vi "Main.vi"() -> ()   [LabVIEW 2018, in "Launcher Main Module.lvlib"]
doc: "This template is based off of the Queued Message Handler design pattern and the Queued Message Handler project template that ships with LabVIEW.\n\nThe main difference is that the queue is private to this module and communication between modules is performed via Broadcast and Request events.\n\nRequest events are wrapped in public API methods and are handled in the Event Handling Loop (EHL) of this VI. Any module can register for Broadcast events sent by this module. The EHL generates messages based on user interface actions.\n\nThe Message Handling Loop (MHL) processes messages generated by the EHL, or by other messages. The messages are string values, so new messages can be added easily to the Message Cases case structure in the MHL. Each message cluster can also provide an optional value for Message Data, which is a variant that can be converted to whatever message-specific data is required.\n_____\nBased on Delacor QMH Project Template 4.2.1.64."
uses:
  Launcher Main Module.lvlib
  <vilib>/Delacor/Delacor QMH/Libraries/Module Admin_class/Delacor_lib_QMH_Module Admin.lvclass
  Module_Controls/Test_Command.ctl
  Module Data--cluster.ctl
  Stop Argument--cluster.ctl
  <vilib>/Delacor/Delacor QMH/Libraries/Message Queue_class/Delacor_lib_QMH_Message Queue.lvclass/Delacor_lib_QMH_Message Queue.ctl
  <vilib>/Delacor/Delacor QMH/Libraries/Module Admin_class/Delacor_lib_QMH_Module Admin.lvclass/Delacor_lib_QMH_Module Admin.ctl
  Module_Controls/Test_Response.ctl
  <vilib>/Utility/miscctls.llb/LVPointTypeDef.ctl
  <vilib>/Delacor/Delacor QMH/Libraries/Message Queue_class/Delacor_lib_QMH_Enqueue Message (Single).vi
  <vilib>/Delacor/Delacor QMH/Libraries/Module Admin_class/Delacor_lib_QMH_Get External Launch.vi
  <vilib>/Utility/error.llb/Error Cluster From Error Code.vi
  <vilib>/ErrorRing/Error Ring.xnode
  <vilib>/Delacor/Delacor QMH/Libraries/Message Queue_class/Delacor_lib_QMH_Message Queue.lvclass
  TCP_Read/TCP_Read.lvlib
  TCP_Write/TCP_Write.lvlib
  TestStand_Control/TestStand_Control.lvlib
panel:
  out "TS_Status":string
  out "command":T1
  out "User_Commands":string
  out "error out":errorcluster
  in  "Module Admin":refnum<class "Delacor_lib_QMH_Module Admin.lvclass">
  out "Status":string
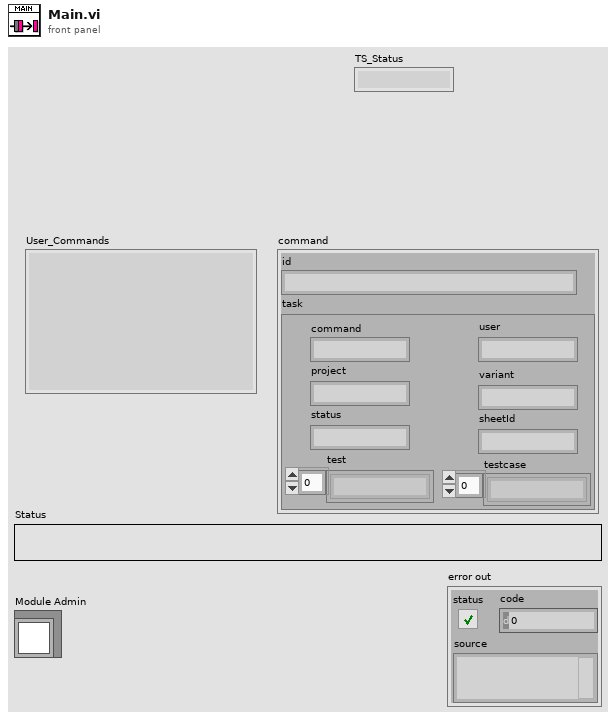
[diagram p1: front panel]
types:
  T1 = typedef "Launcher Main Module.lvlib/Test_Command.ctl" = cluster{"id":string, "task":cluster{"command":string, "project":string, "status":string, "sheetId":string, "test":string[], "user":string, "variant":string, "testcase":string[]}}
  T2 = typedef "Launcher Main Module.lvlib/Request Events--cluster.ctl" = cluster{"Stop Module":refnum<user-event>, "Show Panel":refnum<user-event>, "Hide Panel":refnum<user-event>, "Get Module Execution Status":refnum<user-event>, "Show Diagram":refnum<user-event>}
  T3 = typedef "TestStand_Control.lvlib/Broadcast Events--cluster.ctl" = cluster{"Module Did Init":refnum<user-event>, "Status Updated":refnum<user-event>, "Error Reported":refnum<user-event>, "Module Did Stop":refnum<user-event>, "Update Module Execution Status":refnum<user-event>, "Status":refnum<user-event>}
  T4 = typedef "TCP_Write.lvlib/Broadcast Events--cluster.ctl" = cluster{"Module Did Init":refnum<user-event>, "Status Updated":refnum<user-event>, "Error Reported":refnum<user-event>, "Module Did Stop":refnum<user-event>, "Update Module Execution Status":refnum<user-event>}
  T5 = typedef "TCP_Read.lvlib/Broadcast Events--cluster.ctl" = cluster{"Module Did Init":refnum<user-event>, "Status Updated":refnum<user-event>, "Error Reported":refnum<user-event>, "Module Did Stop":refnum<user-event>, "Update Module Execution Status":refnum<user-event>, "User_Commands":refnum<user-event>}
  T6 = typedef "Launcher Main Module.lvlib/Module Data--cluster.ctl" = cluster{"Status":string}
  T7 = enum32{"invalid lock state", "Not Locked", "Locked (No Password)", "Password-protected"}
  T8 = typedef "Launcher Main Module.lvlib/Stop Argument--cluster.ctl" = cluster{"Origin":string, "Exit via Stop Module Req?":bool, "Wait for Module to stop?":bool}
  T9 = typedef "Launcher Main Module.lvlib/Test_Response.ctl" = cluster{"id":string, "updates":cluster{"status":string}, "command":string, "project":string, "variant":string, "user":string}
  T10 = typedef "LVPointTypeDef.ctl" = cluster{"Horizontal":i16, "Vertical":i16}
  T11 = enum32{"Invalid", "Standard", "Closed", "Hidden", "Minimized", "Maximized"}
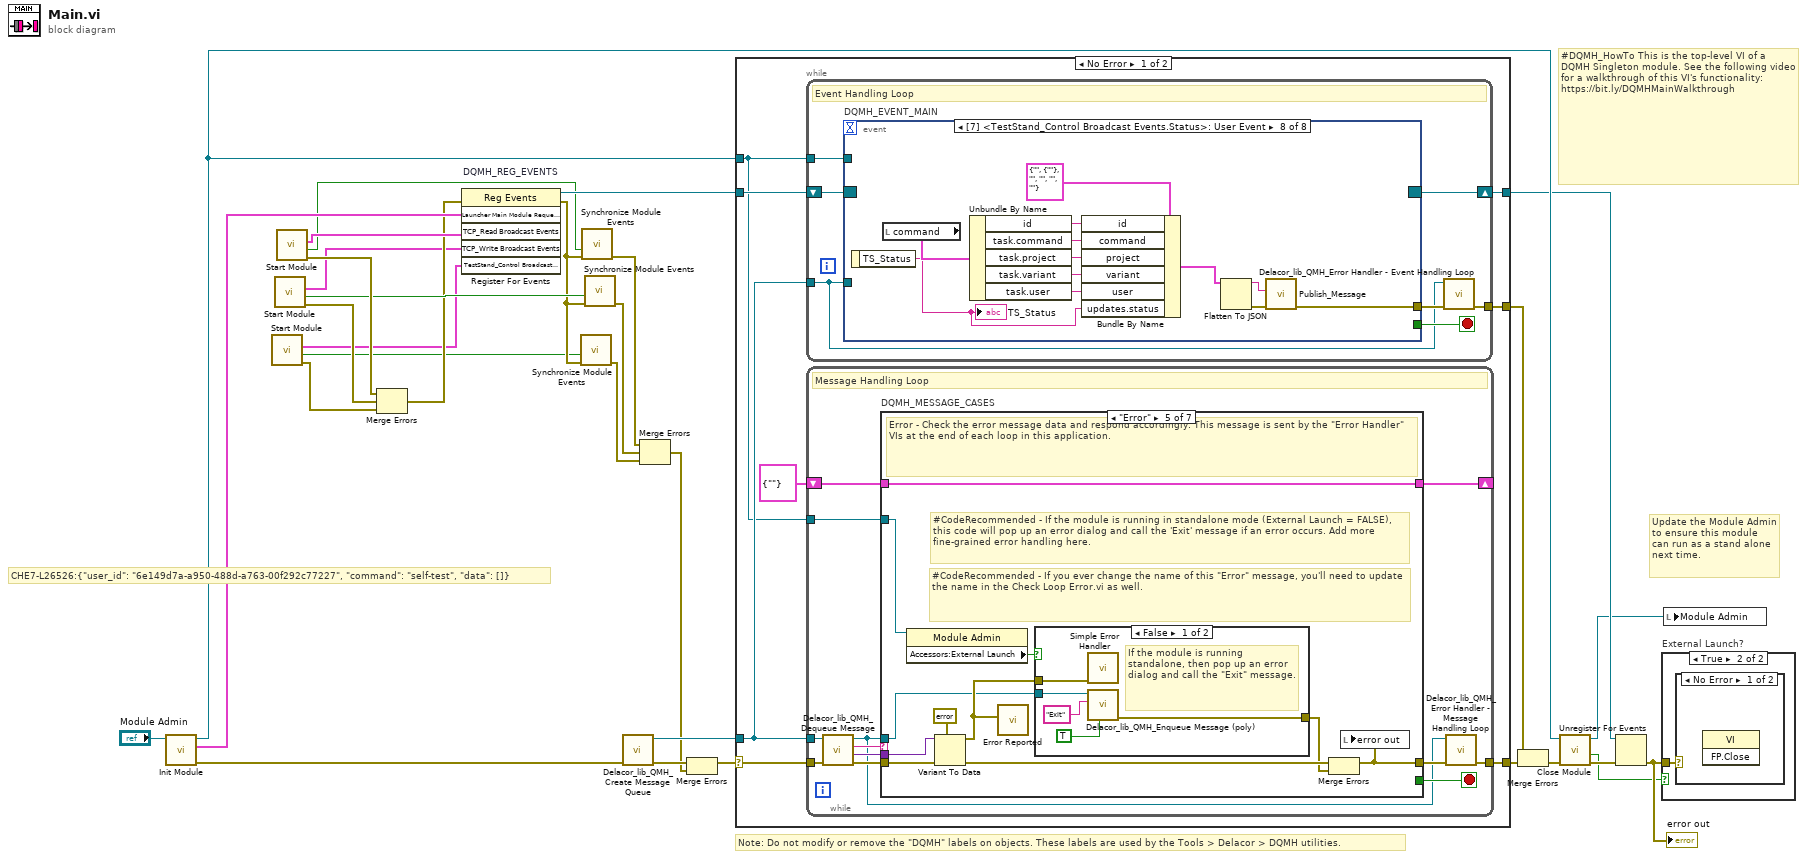
[diagram p0: block diagram]
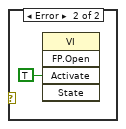
[diagram p3: hidden frame]
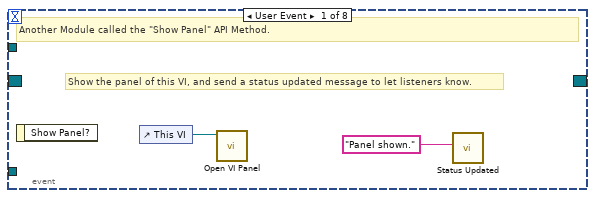
[diagram p4: hidden frame]
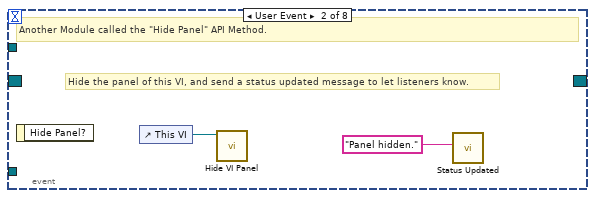
[diagram p5: hidden frame]
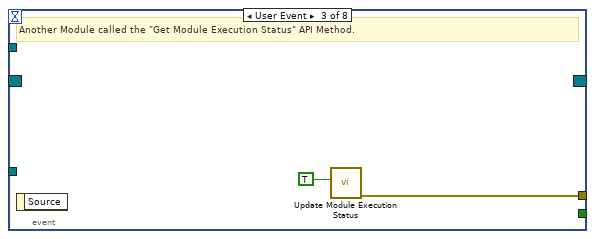
[diagram p6: hidden frame]
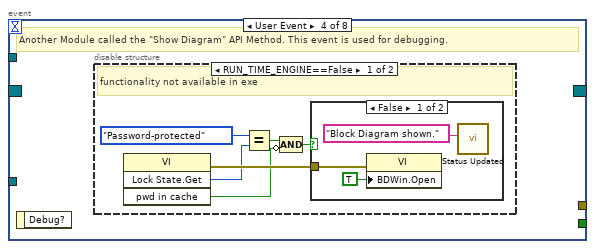
[diagram p7: hidden frame]
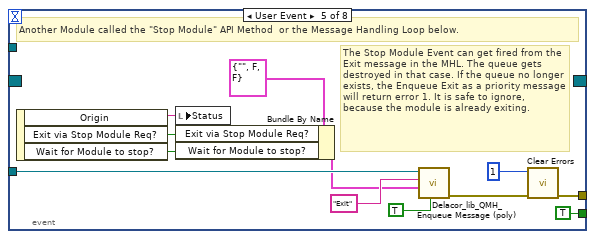
[diagram p10: hidden frame]
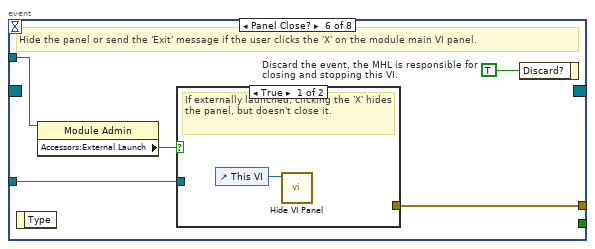
[diagram p11: hidden frame]
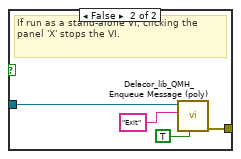
[diagram p12: hidden frame]
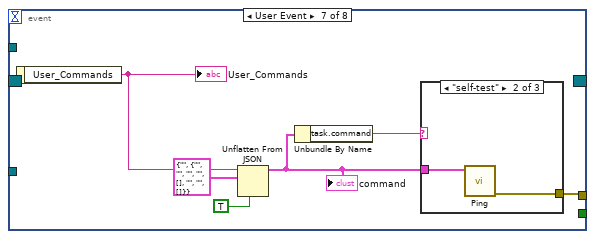
[diagram p13: hidden frame]
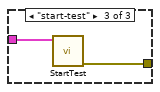
[diagram p15: hidden frame]
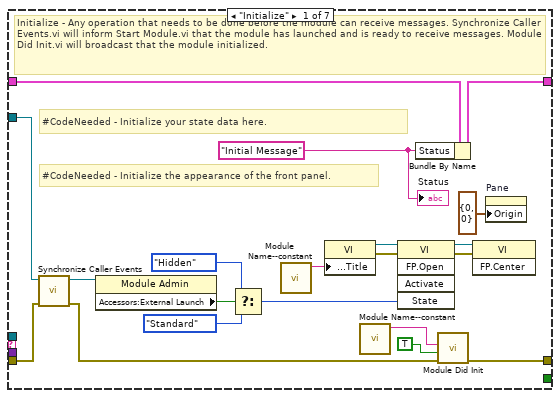
[diagram p16: hidden frame]
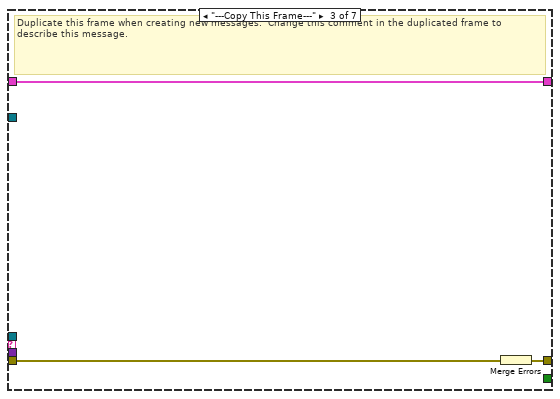
[diagram p18: hidden frame]
diagram:
  # "CHE7-L26526:{\"user_id\": \"6e149d7a-a950-488d-a763-00f292c77227\", \"command\": \"self-test\", \"data\": []}"
  # "#DQMH_HowTo This is the top-level VI of a DQMH Singleton module. See the following video for a walkthrough of this VI's functionality: https://bit.ly/DQMHMainWalkthrough"
  # "Note: Do not modify or remove the \"DQMH\" labels on objects. These labels are used by the Tools > Delacor > DQMH utilities."
  # "Update the Module Admin to ensure this module can run as a stand alone next time."
  n1 = call "Init Module.vi"("Singleton Module Admin in"="Module Admin") -> ("error out"=w30:errorcluster, "Launcher Main Module Request Events"=w20:T2, "Singleton Module Admin out"=w23:refnum<class "Delacor_lib_QMH_Module Admin.lvclass">)  [unwired: 8 in]
  n2 = call "Start Module.vi"() -> ("error out"=w5:errorcluster, "Wait for Event Sync?"=w2:bool, "TestStand_Control Broadcast Events"=w4:T3)  [unwired: 8 in, 1 out]
  n3 = call "Start Module.vi"() -> ("error out"=w6:errorcluster, "Wait for Event Sync?"=w12:bool, "TCP_Write Broadcast Events"=w10:T4)  [unwired: 8 in, 1 out]
  n4 = call "Start Module.vi"() -> ("error out"=w14:errorcluster, "Wait for Event Sync?"=w13:bool, "TCP_Read Broadcast Events"=w15:T5)  [unwired: 8 in, 1 out]
  n5 = Merge Errors(w14, w6, w5) -> (w11:errorcluster)
  n6 = register-events "DQMH_REG_EVENTS"(error in=w11, w20, w15, w10, w4) -> (reference out=w21:refnum<event-registration>, error out=w3:errorcluster)  [unwired: 1 in]
  n7 = call "Synchronize Module Events.vi"("error in (no error)"=w3, "Wait for Event Sync?"=w2) -> ("error out"=w1:errorcluster)  [unwired: 9 in]
  n8 = call "Synchronize Module Events.vi"("error in (no error)"=w3, "Wait for Event Sync?"=w13) -> ("error out"=w9:errorcluster)  [unwired: 9 in]
  n9 = call "Synchronize Module Events.vi"("error in (no error)"=w3, "Wait for Event Sync?"=w12) -> ("error out"=w8:errorcluster)  [unwired: 9 in]
  n10 = call <vilib>:"Delacor_lib_QMH_Create Message Queue.vi"("error in (no error)"=w30) -> ("error out"=w25:errorcluster, "Message Queue"=w19:refnum<class "Delacor_lib_QMH_Message Queue.lvclass">)  [unwired: 9 in]
  n11 = Merge Errors(w9, w8, w1) -> (w7:errorcluster)
  n12 = Merge Errors(w25, w7) -> (w24:errorcluster)
  n13 = case shown="No Error" w24 {
    selector: w24 -> [w37 w197]
    tunnel: [w39 w197] -> w31
    tunnel: [w36 w194] -> w22
    tunnel: w21 -> [w34 w194]
    tunnel: w19 -> [w33 _]
    tunnel: [w38 _] -> w28
    tunnel: w23 -> [w32 w190]
    frame No Error {
      n14 = while {
        tunnel: w33 -> [w40]
        shift-right: [w43] -> w36
        shift-left: w34 -> [w44]
        tunnel: [w45] -> w38
        tunnel: w32 -> [w41]
        stop <- w42 stop-if-true
        # "Event Handling Loop"
        n15 = event "DQMH_EVENT_MAIN" shown="[7] <TestStand_Control Broadcast Events.Status>: User Event" {
          selector: w44 -> [_ _ _ _ _ _ _ _]
          dyn-events: [_ _ _ _ _ _ _ _] -> w43
          timeout: _ -> [_ _ _ _ _ _ _ _]
          tunnel: [_ _ _ _ TRUE ("Discard?") _ _ _] -> w42
          tunnel: w40 -> [_ _ _ _ w69 w76 _ _]
          tunnel: [_ _ w52 _ w72 w78 w88 w105] -> w46
          tunnel: w41 -> [_ _ _ _ _ w75 _ _]
          event User Event {
            # "Show the panel of this VI, and send a status updated message to let listeners know."
            # "Another Module called the \"Show Panel\" API Method."
            n16 = event-data() -> ()  [unwired: 1 in, 1 out]
            n17 = control-ref of="This VI"() -> (w48:refnum<vi>)
            n18 = call "Open VI Panel.vi"("VI"=w48) -> ()  [unwired: 10 in, 1 out]
            n19 = call "Status Updated.vi"("Status"="Panel shown." ("format string")) -> ()  [unwired: 10 in, 1 out]
          }
          event User Event {
            # "Hide the panel of this VI, and send a status updated message to let listeners know."
            # "Another Module called the \"Hide Panel\" API Method."
            n20 = event-data() -> ()  [unwired: 1 in, 1 out]
            n21 = control-ref of="This VI"() -> (w50:refnum<vi>)
            n22 = call "Hide VI Panel.vi"("VI"=w50) -> ()  [unwired: 10 in, 1 out]
            n23 = call "Status Updated.vi"("Status"="Panel hidden." ("format string")) -> ()  [unwired: 10 in, 1 out]
          }
          event User Event {
            # "Another Module called the \"Get Module Execution Status\" API Method."
            n24 = event-data() -> ()  [unwired: 1 in, 1 out]
            n25 = call "Update Module Execution Status.vi"("Running?"=TRUE) -> ("error out"=w52:errorcluster)  [unwired: 10 in]
          }
          event User Event {
            # "Another Module called the \"Show Diagram\" API Method. This event is used for debugging."
            n26 = event-data() -> ()  [unwired: 1 in, 1 out]
            n27 = disable-structure shown="RUN_TIME_ENGINE==False" {
              frame condition #0 (active) {
                # "functionality not available in exe"
                n28 = invoke class="VI" method="Lock State.Get"() -> (error out=w58:errorcluster, "Get Lock State"=w57:T7, "pwd in cache"=w54:bool)  [unwired: 4 in, 1 out]
                n29 = Equal?(x=T7."Password-protected", y=w57) -> (x = y?=w55:bool)
                n30 = Compound Arithmetic op=AND(w55, invert w54) -> (w53:bool)
                n31 = case shown="False" w53 {
                  tunnel: w58 -> [w61 _]
                  frame False {
                    n32 = property class="VI"(error in=w61, "BDWin.Open"=TRUE ("Block Diagram Window:Open")) -> ()  [unwired: 1 in, 2 out]
                    n33 = call "Status Updated.vi"("Status"="Block Diagram shown." ("format string")) -> ()  [unwired: 10 in, 1 out]
                  }
                  frame True {
                    # "Password-protected VI, and the password is not in the cache. Do not show the diagram."
                  }
                }
              }
              frame condition #1 {
              }
            }
          }
          event User Event {
            # "The Stop Module Event can get fired from the Exit message in the MHL. The queue gets destroyed in that case. If the queue no longer exists, the Enqueue Exit as a priority message will return error 1. It is safe to ignore, because the module is already exiting."
            # "Another Module called the \"Stop Module\" API Method  or the Message Handling Loop below."
            n34 = event-data() -> ("Origin"=w68:string, "Exit via Stop Module Req?"=w64:bool, "Wait for Module to stop?"=w63:bool)  [unwired: 1 in]
            n35 = local write "Status"(w68) -> ()
            n36 = Bundle By Name(cluster=T8 {"Origin"="", "Exit via Stop Module Req?"=FALSE, "Wait for Module to stop?"=FALSE} ("Stop Argument"), "Exit via Stop Module Req?"=w64, "Wait for Module to stop?"=w63) -> (w62:T8)
            n37 = call-poly <vilib>:"Delacor_lib_QMH_Enqueue Message (poly).vi"("Priority Message? (F)"=TRUE, "Message Data"=w62, "Message"="Exit", "Message Queue in"=w69) -> ("error out"=w73:errorcluster)  [unwired: 6 in, 1 out]
            n38 = call <vilib>:"Clear Errors.vi"("error in (no error)"=w73, "specific error code to clear (0: all)"=1) -> ("error out"=w72:errorcluster)  [unwired: 4 in, 1 out]
          }
          event Panel Close? {
            w77 = TRUE  # Discard the event, the MHL is responsible for closing and stopping this VI.
            # "Hide the panel or send the 'Exit' message if the user clicks the 'X' on the module main VI panel."
            n39 = event-data() -> ()  [unwired: 1 in, 1 out]
            n40 = property class="Module Admin"(reference=w75) -> ("Accessors:External Launch"=w74:bool)  [unwired: 1 in, 2 out]
            n41 = case shown="True" w74 {
              tunnel: w76 -> [_ w82]
              tunnel: [_ w83] -> w78
              frame True {
                # "If externally launched, clicking the 'X' hides the panel, but doesn't close it."
                n42 = control-ref of="This VI"() -> (w79:refnum<vi>)
                n43 = call "Hide VI Panel.vi"("VI"=w79) -> ()  [unwired: 10 in, 1 out]
              }
              frame False {
                # "If run as a stand-alone VI, clicking the panel 'X' stops the VI."
                n44 = call-poly <vilib>:"Delacor_lib_QMH_Enqueue Message (poly).vi"("Priority Message? (F)"=TRUE, "Message"="Exit", "Message Queue in"=w82) -> ("error out"=w83:errorcluster)  [unwired: 7 in, 1 out]
              }
            }
            n45 = event-data("Discard?"=w77) -> ()  [unwired: 1 in, 1 out]
          }
          event User Event {
            n46 = event-data() -> ("User_Commands"=w84:string)  [unwired: 1 in]
            "User_Commands" <- w84
            n47 = Unflatten From JSON(JSON string=w84, type and defaults=T1 {"id"="", "task"={"command"="", "project"="", "status"="", "sheetId"="", "test"=[], "user"="", "variant"="", "testcase"=[]}} ("test_command"), default null elements? (F)=TRUE) -> (value=w86:T1)  [unwired: 4 in, 1 out]
            "command" <- w86
            n48 = Unbundle By Name(w86) -> ("task.command"=w89:string)
            n49 = case shown="\"self-test\"" w89 {
              tunnel: [_ w91 w93] -> w88
              tunnel: w86 -> [_ w90 w92]
              frame "False", Default {
              }
              frame "self-test" {
                n50 = call "Ping.vi"("test_command"=w90) -> ("error IO"=w91:errorcluster)  [unwired: 10 in]
              }
              frame "start-test" {
                n51 = call "StartTest.vi"("test_command"=w92) -> ("error IO"=w93:errorcluster)  [unwired: 10 in]
              }
            }
          }
          event User Event {
            n52 = event-data() -> ("TS_Status"=w94:string)  [unwired: 1 in]
            "TS_Status" <- w94
            n53 = local read "command"() -> (w100:T1)
            n54 = Unbundle By Name(w100) -> ("id"=w99:string, "task.command"=w98:string, "task.project"=w97:string, "task.variant"=w96:string, "task.user"=w95:string)
            n55 = Bundle By Name(cluster=T9 {"id"="", "updates"={"status"=""}, "command"="", "project"="", "variant"="", "user"=""} ("result"), "id"=w99, "command"=w98, "project"=w97, "variant"=w96, "user"=w95, "updates.status"=w94) -> (w102:T9)
            n56 = Flatten To JSON(anything=w102) -> (JSON string=w103:string, 11:w104:errorcluster)  [unwired: 2 in]
            n57 = call "Publish_Message.vi"("error in (no error)"=w104, "Publish_Message"=w103) -> ("error out"=w105:errorcluster)  [unwired: 9 in]
          }
        }
        n58 = call-dynamic "Delacor_lib_QMH_Error Handler - Event Handling Loop.vi"("error in (no error)"=w46, "Message Queue in"=w40) -> ("dup error in"=w45:errorcluster)  [unwired: 8 in, 1 out]
      }
      n59 = while {
        tunnel: w33 -> [w108]
        shift-right: [w112] -> _
        shift-left: T6 {"Status"=""} ("Data Cluster") -> [w113]
        tunnel: w37 -> [w116]
        tunnel: [w114] -> w39
        tunnel: w32 -> [w106]
        stop <- w111 stop-if-true
        # "Message Handling Loop"
        n60 = call-dynamic "Delacor_lib_QMH_Dequeue Message.vi"("error in (no error)"=w116, "Message Queue in"=w108) -> ("error out"=w115:errorcluster, "Message Data"=w109:variant, "Message"=w110:string, "Message Queue out"=w107:refnum<class "Delacor_lib_QMH_Message Queue.lvclass">)  [unwired: 6 in]
        n61 = case "DQMH_MESSAGE_CASES" shown="\"Error\"" w110 {
          selector: w110 -> [_ _ _ _ _ _ w177]
          tunnel: w107 -> [_ _ _ _ w147 w169 _]
          tunnel: w115 -> [w135 w139 w142 w144 w154 w175 w179]
          tunnel: [w133 w139 w141 w144 w150 w172 w180] -> w117
          tunnel: w113 -> [w124 w138 w140 w143 w149 w168 w178]
          tunnel: [w123 w138 w140 w143 w149 w168 w178] -> w112
          tunnel: [_ _ _ _ _ w167 _] -> w111
          tunnel: w109 -> [_ _ _ _ w148 w166 _]
          tunnel: w106 -> [w125 _ _ _ w146 w161 _]
          frame "Initialize" {
            w118 = "Initial Message" ("Initial Message")
            # "#CodeNeeded - Initialize the appearance of the front panel."
            # "#CodeNeeded - Initialize your state data here."
            # "Initialize - Any operation that needs to be done before the module can receive messages. Synchronize Caller Events.vi will inform Start Module.vi that the module has launched and is ready to receive messages. Module Did Init.vi will broadcast that the module initialized."
            n62 = call "Synchronize Caller Events.vi"("error in (no error)"=w135, "Singleton Module Admin in"=w125) -> ("error out"=w134:errorcluster, "Singleton Module Admin out"=w120:refnum<class "Delacor_lib_QMH_Module Admin.lvclass">)  [unwired: 8 in]
            n63 = property class="Module Admin"(reference=w120) -> ("Accessors:External Launch"=w129:bool)  [unwired: 1 in, 2 out]
            n64 = Select(t=T11."Hidden" ("State"), s=w129, f=T11."Standard" ("State")) -> (s? t:f=w126:T11)
            n65 = call "Module Name--constant.vi"() -> ("Module Name"=w132:string)  [unwired: 11 in]
            n66 = property class="VI"("Front Panel.Title"=w132) -> (reference out=w131:refnum<vi>, error out=w137:errorcluster)  [unwired: 2 in]
            n67 = call "Module Name--constant.vi"() -> ("Module Name"=w121:string)  [unwired: 11 in]
            n68 = invoke class="VI" method="FP.Open"(reference=w131, error in=w137, "State"=w126) -> (reference out=w130:refnum<vi>, error out=w136:errorcluster)  [unwired: 2 in, 3 out]
            n69 = Bundle By Name(cluster=w124, "Status"=w118) -> (w123:T6)
            n70 = call "Module Did Init.vi"("error in (no error)"=w134, "Initialized?"=TRUE, "Origin"=w121) -> ("error out"=w133:errorcluster)  [unwired: 8 in]
            n71 = invoke class="VI" method="FP.Center"(reference=w130, error in=w136) -> ()  [unwired: 1 in, 3 out]
            n72 = property on="Pane" class="Pane"("Origin"=T10 {"Horizontal"=0, "Vertical"=0}) -> ()  [unwired: 2 in, 2 out]
            "Status" <- w118
          }
          frame "--- Module Specific ---" {
            # "Separator -- The following cases handle messages specific to this Module."
          }
          frame "---Copy This Frame---" {
            # "Duplicate this frame when creating new messages.  Change this comment in the duplicated frame to describe this message."
            n73 = Merge Errors(w142) -> (w141:errorcluster)
          }
          frame "--- Exit and Error Handling---" {
            # "Separator - The following cases handle errors and exit messages."
          }
          frame "Error" {
            # "#CodeRecommended - If you ever change the name of this \"Error\" message, you'll need to update the name in the Check Loop Error.vi as well."
            # "#CodeRecommended - If the module is running in standalone mode (External Launch = FALSE), this code will pop up an error dialog and call the 'Exit' message if an error occurs. Add more fine-grained error handling here."
            # "Error - Check the error message data and respond accordingly. This message is sent by the \"Error Handler\" VIs at the end of each loop in this application."
            n74 = property class="Module Admin"(reference=w146) -> ("Accessors:External Launch"=w145:bool)  [unwired: 1 in, 2 out]
            n75 = Variant To Data(error in=w154, type=errorcluster {"status"=FALSE, "code"=0, "source"=""} ("error constant"), Variant=w148) -> (data=w155:errorcluster, error out=w152:errorcluster)
            n76 = call "Error Reported.vi"("Error"=w155) -> ()  [unwired: 10 in, 1 out]
            n77 = case shown="False" w145 {
              tunnel: [w160 _] -> w151
              tunnel: w147 -> [w158 _]
              tunnel: w155 -> [w159 _]
              frame False {
                # "If the module is running standalone, then pop up an error dialog and call the \"Exit\" message."
                n78 = call <vilib>:"Simple Error Handler.vi"("error in (no error)"=w159) -> ()  [unwired: 4 in, 5 out]
                n79 = call-poly <vilib>:"Delacor_lib_QMH_Enqueue Message (poly).vi"("Priority Message? (F)"=TRUE, "Message"="Exit", "Message Queue in"=w158) -> ("error out"=w160:errorcluster)  [unwired: 7 in, 1 out]
              }
              frame True {
                # "If the module was launched externally, calling the Error Reported broadcast VI is the only action performed by the \"Error\" message. The module's caller can then process the error appropriately."
              }
            }
            n80 = Merge Errors(w152, w151) -> (w150:errorcluster)
            n81 = local write "error out"(w150) -> ()
          }
          frame "Exit" {
            w165 = 91  # 91: not all Exit messages will have an argument
            w167 = TRUE  # Stop the VI
            # "Release the message queue reference"
            # "#CodeNeeded - Add any required cleanup code here"
            # "Exit - Exit the application."
            n82 = Variant To Data(error in=w175, type=T8 {"Origin"="", "Exit via Stop Module Req?"=FALSE, "Wait for Module to stop?"=FALSE} ("Stop Argument"), Variant=w166) -> (data=w163:T8, error out=w171:errorcluster)
            n83 = call <vilib>:"Clear Errors.vi"("error in (no error)"=w171, "specific error code to clear (0: all)"=w165) -> ("error out"=w174:errorcluster)  [unwired: 4 in, 1 out]
            n84 = control-ref of="This VI"() -> (w162:refnum<vi>)
            n85 = call-dynamic "Delacor_lib_QMH_Release Message Queue.vi"("error in (no error)"=w174, "Message Queue"=w169) -> ("error out"=w173:errorcluster)  [unwired: 9 in]
            n86 = call "Handle Exit.vi"("Stop Argument"=w163, "Admin in"=w161, "VI reference"=w162) -> ("error out"=w170:errorcluster)  [unwired: 7 in, 1 out]
            n87 = Merge Errors(w173, w170) -> (w172:errorcluster)
            n88 = call "Stop Module.vi"() -> ()  [unwired: 11 in, 1 out]
            n89 = call "Stop Module.vi"() -> ()  [unwired: 11 in, 1 out]
            n90 = call "Stop Module.vi"() -> ()  [unwired: 11 in, 1 out]
          }
          frame Default {
            # "'Default' case only runs if there is a message that isn't defined in any of the other cases.  Output a programming error."
            n91 = call "Module Name--constant.vi"() -> ("Module Name"=w176:string)  [unwired: 11 in]
            n92 = xnode "Error Ring"("parameter 0"=w177, "parameter 1"=w176) -> ("error out"=w181:errorcluster)
            n93 = Merge Errors(w179, w181) -> (w180:errorcluster)
          }
        }
        n94 = call-dynamic "Delacor_lib_QMH_Error Handler - Message Handling Loop.vi"("error in (no error)"=w117, "Message Queue in"=w107) -> ("dup error in"=w114:errorcluster)  [unwired: 8 in, 1 out]
      }
    }
    frame Error {
      # "Synchronize Caller Events.vi will inform Start Module.vi that the module has launched and will let the code calling Start Module.vi register for broadcasts and would permit the caller receive the broadcast that an error occurred at launch time."
      n95 = call "Synchronize Caller Events.vi"("Singleton Module Admin in"=w190) -> ("error out"=w195:errorcluster)  [unwired: 9 in, 1 out]
      n96 = call "Module Name--constant.vi"() -> ("Module Name"=w193:string)  [unwired: 11 in]
      n97 = Format Into String(format string="An error occurred during initialization. %s is no longer running.", w193) -> (resulting string=w191:string)  [unwired: 2 in, 1 out]
      n98 = Merge Errors(w197, w195) -> (w196:errorcluster)
      n99 = call "Error Reported.vi"("Additional Information"=w191, "Error"=w196) -> ()  [unwired: 9 in, 1 out]
    }
  }
  n100 = Merge Errors(w28, w31) -> (w27:errorcluster)
  n101 = call "Close Module.vi"("error in (no error)"=w27, "Module Admin in"=w23) -> ("error out"=w29:errorcluster, "External Launch"=w16:bool, "Module Admin out"=w17:refnum<class "Delacor_lib_QMH_Module Admin.lvclass">)  [unwired: 7 in]
  n102 = Unregister For Events(event registration refnum=w22, error in=w29) -> (error out=w26:errorcluster)
  "error out" <- w26
  n103 = case "External Launch?" shown="True" w16 {
    tunnel: w26 -> [_ w198]
    frame False {
    }
    frame True {
      n104 = case shown="No Error" w198 {
        frame No Error {
          n105 = invoke class="VI" method="FP.Close"() -> ()  [unwired: 3 in, 3 out]
        }
        frame Error {
          n106 = invoke class="VI" method="FP.Open"("Activate"=TRUE ("Activate?")) -> ()  [unwired: 4 in, 5 out]
        }
      }
    }
  }
  n107 = local write "Module Admin"(w17) -> ()
